vi "MH_CalcDeltaTNeg_EB.vi"(0 "WinDelta":i32, 1 "TrueTime":u64, 2 "WIndowW":i32, 4 "DBuffSize":i32=10, 5 "Data In":u64[](array[numeric]), 7 "DeltasBuffer":i32[](array[numeric]), 9 "Deltaindex":i32, 11 "error In":errorcluster, 12 "WinIndex":i32, 13 "queue out":refnum<queue>) -> (3 "WinDelta Out":i32, 6 "DeltasBufferOut":i32[](array[numeric]), 8 "DeltaIndexOut":i32, 10 "NewDelta":bool, 14 "WinIndexOut":i32, 15 "Error Out":errorcluster caption="error Out")   [LabVIEW 2019]
uses:
  <userlib>/MultiHarp150/T2Lib/MH_T2DeltaQMessage.ctl
panel:
  in  "Buffsize":i32
  # "here"
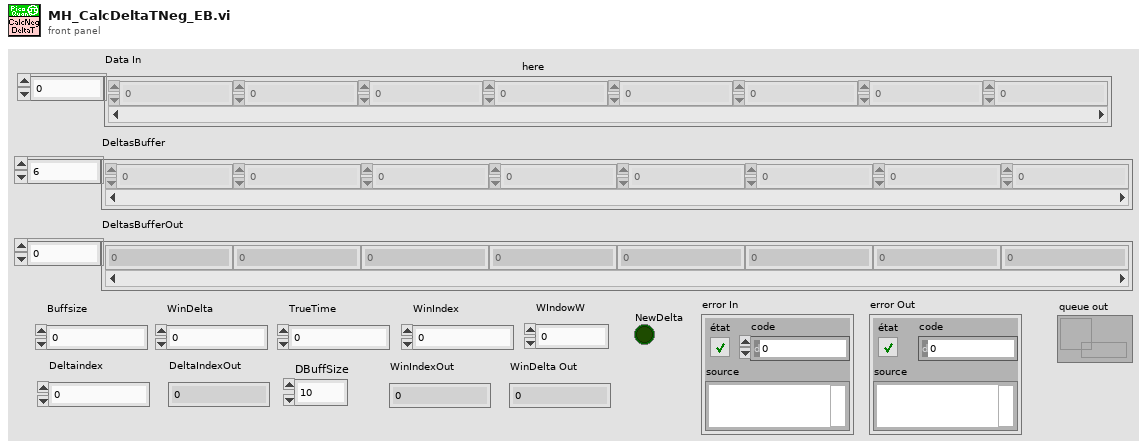
[diagram p1: front panel]
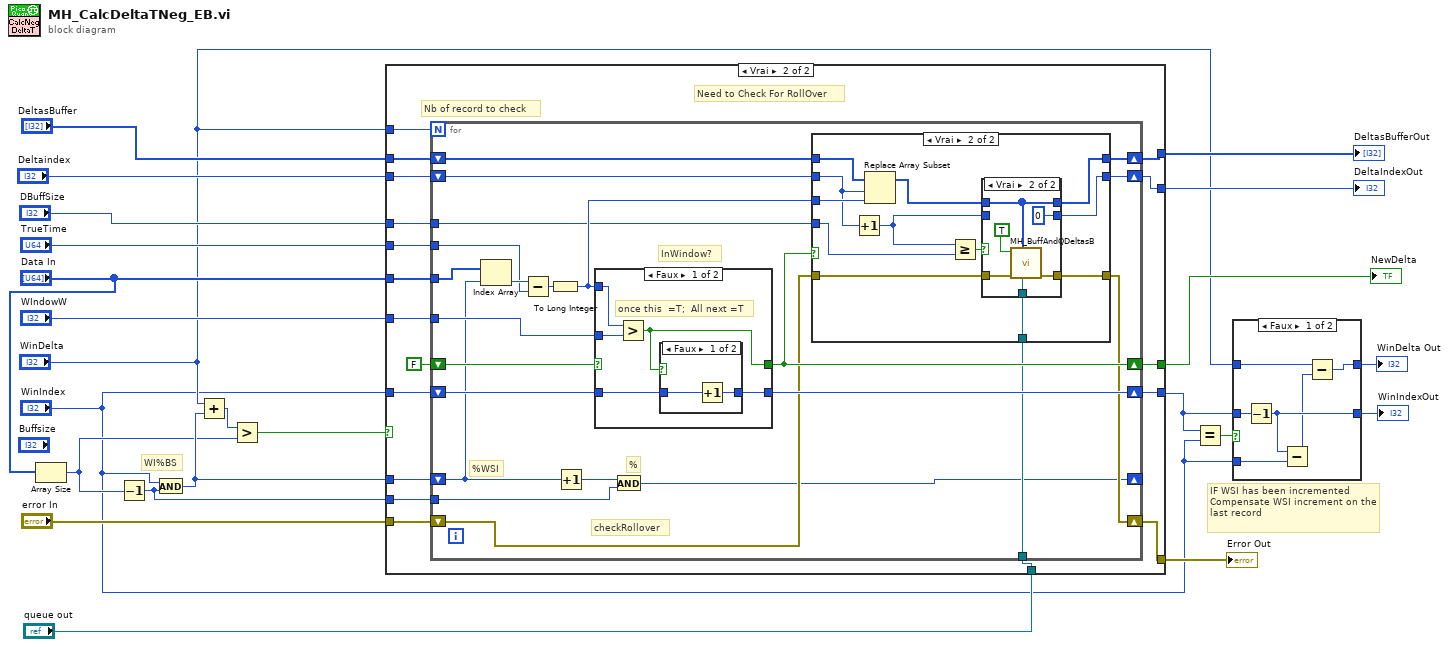
[diagram p0: block diagram]
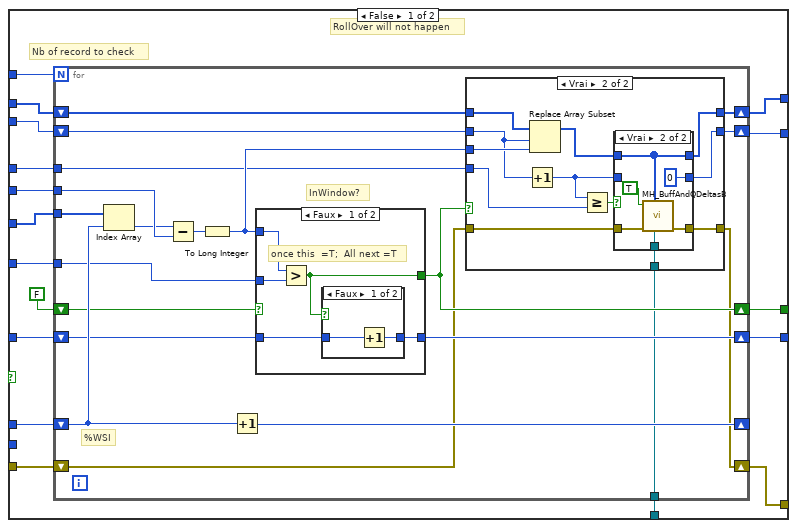
[diagram p2: hidden frame]
diagram:
  # "WI%BS"
  # "IF WSI has been incremented\nCompensate WSI increment on the last record"
  n1 = Array Size(array="Data In") -> (size(s)=w6:i32)
  n2 = Decrement(x=w6) -> (x-1=w8:i32)
  n3 = And(x="WinIndex", y=w8) -> (x .and. y?=w20:i32)
  n4 = Add(x="WinDelta", y=w20) -> (x+y=w19:i32)
  n5 = Greater?(x=w19, y=w6) -> (0:w18:bool)
  n6 = case shown="Vrai" w18 {
    tunnel: "Data In" -> [w40 w112]
    tunnel: "TrueTime" -> [w39 w111]
    tunnel: "WIndowW" -> [w38 w110]
    tunnel: [w37 w109] -> w22
    tunnel: "WinIndex" -> [w35 w107]
    tunnel: [w34 w106] -> w5
    tunnel: "WinDelta" -> [w33 w98]
    tunnel: w20 -> [w32 w105]
    tunnel: "DeltasBuffer" -> [w31 w104]
    tunnel: "Deltaindex" -> [w30 w103]
    tunnel: [w28 w102] -> w17
    tunnel: [w29 w101] -> w16
    tunnel: "DBuffSize" -> [w27 w97]
    tunnel: "queue out" -> [w26 w96]
    tunnel: "error In" -> [w25 w100]
    tunnel: [w24 w99] -> w10
    tunnel: w8 -> [_ w95]
    frame False {
      # "RollOver will not happen"
      # "Nb of record to check"
      n7 = for {
        N: w33 -> [_]
        tunnel: w40 -> [w60]
        tunnel: w39 -> [w42]
        shift-right: [w54] -> w34
        shift-left: w35 -> [w55]
        shift-right: [w53] -> _
        shift-left: w32 -> [w58]
        tunnel: w38 -> [w57]
        shift-right: [w47] -> w37
        shift-left: FALSE -> [w56]
        shift-right: [w49] -> w28
        shift-left: w31 -> [w52]
        shift-right: [w48] -> w29
        shift-left: w30 -> [w51]
        tunnel: w27 -> [w46]
        tunnel: w26 -> [w45]
        shift-right: [w44] -> w24
        shift-left: w25 -> [w43]
        # "InWindow?"
        # "%WSI"
        n8 = Index Array(array=w60, index=w58) -> (element=w41:u64)
        n9 = Subtract(x=w41, y=w42) -> (x-y=w59:u64)
        n10 = To Long Integer(number=w59) -> (32bit integer=w50:i32)
        n11 = Increment(x=w58) -> (x+1=w53:i32)
        n12 = case shown="Faux" w56 {
          selector: w56 -> [_ w93]
          tunnel: w50 -> [w89 _]
          tunnel: w57 -> [w88 _]
          tunnel: [w86 w93] -> w47
          tunnel: w55 -> [w87 w94]
          tunnel: [w85 w94] -> w54
          frame False {
            # "once this  =T;  All next =T"
            n13 = Greater?(x=w89, y=w88) -> (0:w86:bool)
            n14 = case shown="Faux" w86 {
              tunnel: [w90 w92] -> w85
              tunnel: w87 -> [w91 w92]
              frame False {
                n15 = Increment(x=w91) -> (x+1=w90:i32)
              }
              frame True {
              }
            }
          }
          frame True {
          }
        }
        n16 = case shown="Vrai" w47 {
          tunnel: w52 -> [w63 w74]
          tunnel: w50 -> [_ w75]
          tunnel: w51 -> [w62 w73]
          tunnel: [w62 w66] -> w48
          tunnel: [w63 w64] -> w49
          tunnel: w46 -> [_ w68]
          tunnel: w45 -> [_ w71]
          tunnel: [w61 w70] -> w44
          tunnel: w43 -> [w61 w69]
          frame False {
          }
          frame True {
            n17 = Increment(x=w73) -> (x+1=w67:i32)
            n18 = Replace Array Subset(array=w74, new element=w75, index=w73) -> (w65:i32[])
            n19 = Greater Or Equal?(x=w67, y=w68) -> (x >= y?=w72:bool)
            n20 = case shown="Vrai" w72 {
              tunnel: w71 -> [_ w84]
              tunnel: [w78 w83] -> w70
              tunnel: w69 -> [w78 w82]
              tunnel: w65 -> [w76 w80]
              tunnel: w67 -> [w77 _]
              tunnel: [w77 0] -> w66
              tunnel: [w76 w80] -> w64
              frame False {
              }
              frame True {
                n21 = call <userlib>:"MH_BuffAndQDeltasB.vi"("queue out"=w84, "DeltasBuffer"=w80, "erroIn"=w82, "Limit Queue SIze"=TRUE) -> ("error out"=w83:errorcluster)  [unwired: 7 in]
              }
            }
          }
        }
      }
    }
    frame True {
      # "Need to Check For RollOver"
      # "Nb of record to check"
      n22 = for {
        N: w98 -> [_]
        tunnel: w112 -> [w134]
        tunnel: w111 -> [w117]
        shift-right: [w130] -> w106
        shift-left: w107 -> [w131]
        shift-right: [w114] -> _
        shift-left: w105 -> [w116]
        tunnel: w110 -> [w133]
        shift-right: [w125] -> w109
        shift-left: FALSE -> [w132]
        shift-right: [w128] -> w102
        shift-left: w104 -> [w126]
        shift-right: [w127] -> w101
        shift-left: w103 -> [w124]
        shift-right: [w121] -> w99
        shift-left: w100 -> [w122]
        tunnel: w97 -> [w120]
        tunnel: w96 -> [w119]
        tunnel: w95 -> [w115]
        # "%"
        # "InWindow?"
        # "checkRollover"
        # "%WSI"
        n23 = Index Array(array=w134, index=w116) -> (element=w118:u64)
        n24 = Subtract(x=w118, y=w117) -> (x-y=w129:u64)
        n25 = To Long Integer(number=w129) -> (32bit integer=w123:i32)
        n26 = Increment(x=w116) -> (x+1=w113:i32)
        n27 = case shown="Faux" w132 {
          selector: w132 -> [_ w167]
          tunnel: w123 -> [w163 _]
          tunnel: w133 -> [w162 _]
          tunnel: [w161 w167] -> w125
          tunnel: w131 -> [w159 w168]
          tunnel: [w160 w168] -> w130
          frame False {
            # "once this  =T;  All next =T"
            n28 = Greater?(x=w163, y=w162) -> (0:w161:bool)
            n29 = case shown="Faux" w161 {
              tunnel: [w164 w166] -> w160
              tunnel: w159 -> [w165 w166]
              frame False {
                n30 = Increment(x=w165) -> (x+1=w164:i32)
              }
              frame True {
              }
            }
          }
          frame True {
          }
        }
        n31 = And(x=w113, y=w115) -> (x .and. y?=w114:i32)
        n32 = case shown="Vrai" w125 {
          tunnel: w126 -> [w137 w148]
          tunnel: w123 -> [_ w149]
          tunnel: w124 -> [w136 w147]
          tunnel: [w136 w146] -> w127
          tunnel: [w137 w138] -> w128
          tunnel: w122 -> [w135 w144]
          tunnel: [w135 w143] -> w121
          tunnel: w120 -> [_ w141]
          tunnel: w119 -> [_ w140]
          frame False {
          }
          frame True {
            n33 = Increment(x=w147) -> (x+1=w142:i32)
            n34 = Replace Array Subset(array=w148, new element=w149, index=w147) -> (w139:i32[])
            n35 = Greater Or Equal?(x=w142, y=w141) -> (x >= y?=w145:bool)
            n36 = case shown="Vrai" w145 {
              tunnel: w140 -> [_ w158]
              tunnel: [w152 w157] -> w143
              tunnel: w144 -> [w152 w156]
              tunnel: w139 -> [w150 w154]
              tunnel: w142 -> [w151 _]
              tunnel: [w151 0] -> w146
              tunnel: [w150 w154] -> w138
              frame False {
              }
              frame True {
                n37 = call <userlib>:"MH_BuffAndQDeltasB.vi"("queue out"=w158, "DeltasBuffer"=w154, "erroIn"=w156, "Limit Queue SIze"=TRUE) -> ("error out"=w157:errorcluster)  [unwired: 7 in]
              }
            }
          }
        }
      }
    }
  }
  "NewDelta" <- w22
  "DeltasBufferOut" <- w17
  "DeltaIndexOut" <- w16
  "Error Out" <- w10
  n38 = Equal?(x=w5, y="WinIndex") -> (x = y?=w4:bool)
  n39 = case shown="Faux" w4 {
    tunnel: [w171 w176] -> w21
    tunnel: w5 -> [w172 w176]
    tunnel: "WinDelta" -> [w174 w175]
    tunnel: [w170 w175] -> w2
    tunnel: "WinIndex" -> [w173 _]
    frame False {
      n40 = Decrement(x=w172) -> (x-1=w171:i32)
      n41 = Subtract(x=w171, y=w173) -> (x-y=w169:i32)
      n42 = Subtract(x=w174, y=w169) -> (x-y=w170:i32)
    }
    frame True {
    }
  }
  "WinIndexOut" <- w21
  "WinDelta Out" <- w2
